vi "1D Convolution (CDB).vi"(9 "algorithm":enum32{"direct", "frequency domain"}(ring)=enum."frequency domain", 10 "Y":cdb[](array[numeric]), 11 "X":cdb[](array[numeric])) -> (0 "error":i32, 3 "X * Y":cdb[](array[numeric]))   [LabVIEW 2020, in "NI_AALPro.lvlib"]
doc: "Computes the convolution of the input sequences <B>X</B> and <B>Y</B>. Wire data to the <B>X</B> and <B>Y</B> inputs to determine the polymorphic instance to use or manually select the instance."
uses:
  NI_AALPro.lvlib
  <resource>/lvanlys.dll
panel:
  # "1D Convolution (CDB)"
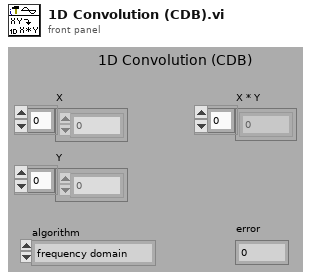
[diagram p1: front panel]
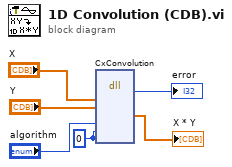
[diagram p0: block diagram]
diagram:
  w5 = 0 ("ConvOrCorr")
  n1 = dll-call lib="C:/Program Files (x86)/National Instruments/LabVIEW 2020/resource/lvanlys.*" fn="CxConvolution"("X"="X", "Y"="Y", "domain"="algorithm", "ConvOrCorr"=w5, "norm"=w5) -> (→"error":i32, "X * Y"=→"X * Y":cdb[])  [unwired: 9 in, 2 out]
